vi "Driver.vi"(8 "error in (no error)":errorcluster, 11 "XBoxController":refnum<class "XBoxController.lvclass">) -> (0 "error out":errorcluster)   [LabVIEW 2013]
uses:
  XboxController/XBoxController.lvclass
  DriverXBoxController/DriverXBoxController.lvclass
  DriveMotors/DriveMotors.lvclass
  Shifter/Shifter.lvclass
  XboxController/XBoxController.lvclass/XBoxController.ctl
  Robot Global Data.vi
  <vilib>/Rock Robotics/WPI/Joystick/WPI_JoystickGet.vi
  Commands/DM-SetPower-Command/DM-SetPower-Command.lvclass
panel:
  out "RightPower 2":dbl
  out "LeftPower 2":dbl
  in  "Square Inputs?":bool
  in  "Arcade(T) or Tank(F)":bool=TRUE
  out "Xbox Triggers":T1 {"Right Trigger" scale=0.0..1.0; "Left Trigger" scale=0.0..1.0}
  out "LeftJoystick.Right":dbl(slide) scale=-1.0..1.0
  out "LeftJoystick.Forward":dbl(slide) scale=-1.0..1.0
  out "RightPower":dbl(slide) scale=-1.0..1.0
  out "LeftPower":dbl(slide) scale=-1.0..1.0
  in  "Semaphore Timeout":i32=-1
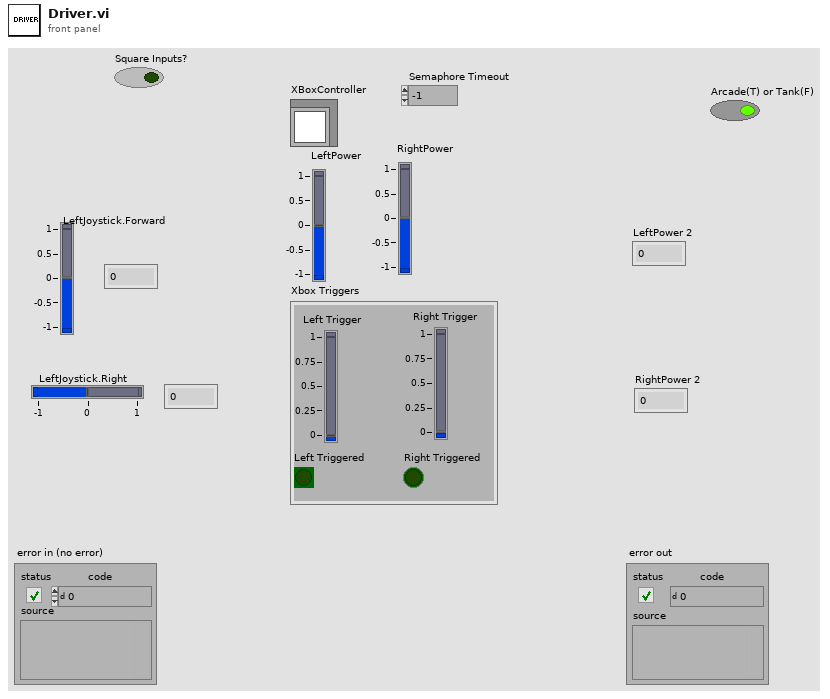
[diagram p1: front panel]
types:
  T1 = cluster{"Left Trigger":dbl, "Right Trigger":dbl, "Left Triggered":bool, "Right Triggered":bool}
  T2 = typedef "XBoxController.lvclass/Xbox Buttons.ctl" = cluster{"RightBumper":bool, "Left Bumper":bool, "Left Joy Down":bool, "Right Joy Down":bool, "Back":bool, "Start":bool, "D-Pad Left":bool, "D-Pad Right":bool, "Y":bool, "B":bool, "A":bool, "X":bool}
  T3 = cluster{"LeftJoystick":cluster{"Forward":dbl, "Right":dbl}, "RightJoystick":cluster{"Forward":dbl, "Right":dbl}}
  T4 = typedef "Semaphore RefNum" = refnum<k1>
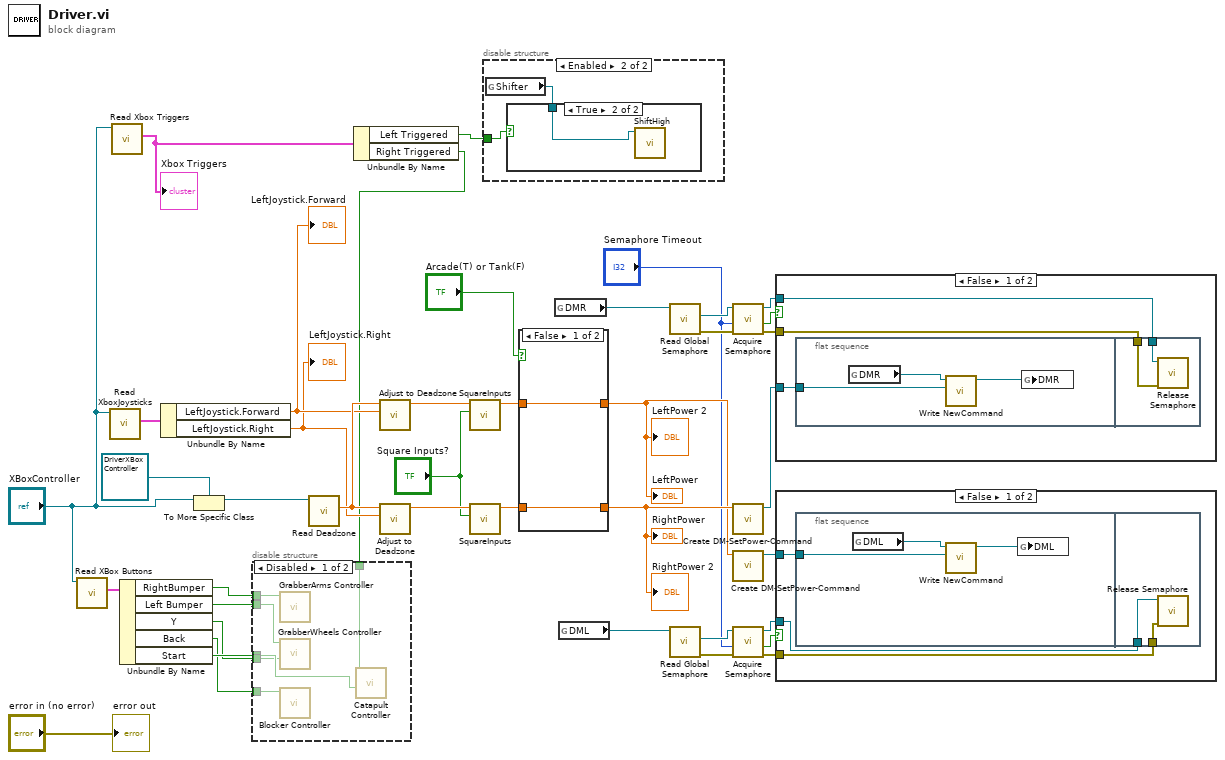
[diagram p0: block diagram]
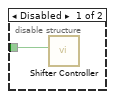
[diagram p2: hidden frame]
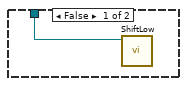
[diagram p3: hidden frame]
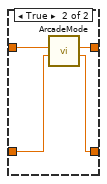
[diagram p5: hidden frame]
diagram:
  n1 = call "Read XBox Buttons.vi"("XBoxController in"="XBoxController") -> ("XBox Buttons"=w8:T2)  [unwired: 8 in, 2 out]
  n2 = call-dynamic "Read XboxJoysticks.vi"("XBoxController in"="XBoxController") -> ("XboxJoysticks"=w40:T3)  [unwired: 8 in, 2 out]
  n3 = call-dynamic "Read Xbox Triggers.vi"("XBoxController in"="XBoxController") -> ("Xbox Triggers"=w38:T1)  [unwired: 8 in, 2 out]
  "Xbox Triggers" <- w38
  n4 = Unbundle By Name(w8) -> ("RightBumper"=w7:bool, "Left Bumper"=w6:bool, "Y"=w4:bool, "Back"=w3:bool, "Start"=w5:bool)
  n5 = Unbundle By Name(w40) -> ("LeftJoystick.Forward"=w11:dbl, "LeftJoystick.Right"=w10:dbl)
  "LeftJoystick.Forward" <- w11
  "LeftJoystick.Right" <- w10
  n6 = To More Specific Class(target class=refnum<class "DriverXBoxController.lvclass"> refnum ("DriverXBoxController.lvclass"), reference="XBoxController") -> (specific class reference=w19:refnum<class "DriverXBoxController.lvclass">)  [unwired: 1 in, 1 out]
  n7 = call-dynamic "Read Deadzone.vi"("DriverXBoxController in"=w19) -> ("Deadzone"=w18:dbl)  [unwired: 8 in, 2 out]
  n8 = Unbundle By Name(w38) -> ("Left Triggered"=w2:bool, "Right Triggered"=w1:bool)
  n9 = disable-structure shown="Disabled" {
    disable-tunnel: w7 -> [w46 _]
    disable-tunnel: w6 -> [w45 _]
    disable-tunnel: w5 -> [w44 _]
    disable-tunnel: w4 -> [w43 _]
    disable-tunnel: w3 -> [w42 _]
    disable-tunnel: w1 -> [w41 _]
    frame Disabled {
      n10 = call "GrabberArms Controller.vi"("Extend GrabberArms"=w46) -> ()  [unwired: 10 in, 1 out]
      n11 = call "GrabberWheels Controller.vi"("GW Spit Out"=w43, "GW Full Speed Pickup"=w45) -> ()  [unwired: 9 in, 1 out]
      n12 = call "Blocker Controller.vi"("Blocker Toggle"=w42) -> ()  [unwired: 11 in]
      n13 = call "Catapult Controller.vi"("De-energize w/out Re-energizing"=w44, "Catapult Trigger"=w41) -> ()  [unwired: 9 in, 1 out]
    }
    frame Enabled {
    }
  }
  n14 = call "Adjust to Deadzone.vi"("Axis Value"=w11, "Deadzone"=w18) -> ("Adjusted Axis Value"=w16:dbl)  [unwired: 9 in]
  n15 = call "Adjust to Deadzone.vi"("Axis Value"=w10, "Deadzone"=w18) -> ("Adjusted Axis Value"=w14:dbl)  [unwired: 9 in]
  n16 = call "SquareInputs.vi"("Square Inputs?"="Square Inputs?", "AxisValueIn"=w16) -> ("AxisValueOut"=w15:dbl)  [unwired: 9 in]
  n17 = call "SquareInputs.vi"("Square Inputs?"="Square Inputs?", "AxisValueIn"=w14) -> ("AxisValueOut"=w13:dbl)  [unwired: 9 in]
  n18 = disable-structure shown="Enabled" {
    disable-tunnel: w2 -> [w47 w48]
    frame Disabled {
      n19 = call "Shifter Controller.vi"("ShiftHigh"=w47) -> ()  [unwired: 11 in]
    }
    frame Enabled {
      n20 = global read "Robot Global Data.vi" "Shifter"() -> (w49:refnum<class "Shifter.lvclass">)
      n21 = case shown="True" w48 {
        tunnel: w49 -> [w50 w51]
        frame False {
          n22 = call-dynamic "ShiftLow.vi"("Shifter in"=w50) -> ()  [unwired: 9 in, 2 out]
        }
        frame True {
          n23 = call-dynamic "ShiftHigh.vi"("Shifter in"=w51) -> ()  [unwired: 9 in, 2 out]
        }
      }
    }
  }
  n24 = case shown="False" "Arcade(T) or Tank(F)" {
    tunnel: [w52 w57] -> w37
    tunnel: [w53 w56] -> w24
    tunnel: w15 -> [w53 w55]
    tunnel: w13 -> [w52 w54]
    frame False {
    }
    frame True {
      n25 = call "ArcadeMode.vi"("RightPower"=w54, "ForwardPower"=w55) -> ("RightPower"=w57:dbl, "LeftPower"=w56:dbl)  [unwired: 8 in]
    }
  }
  "LeftPower" <- w24
  "RightPower" <- w37
  "LeftPower 2" <- w24
  "RightPower 2" <- w37
  n26 = global read "Robot Global Data.vi" "DMR"() -> (w35:refnum<class "DriveMotors.lvclass">)
  n27 = global read "Robot Global Data.vi" "DML"() -> (w31:refnum<class "DriveMotors.lvclass">)
  n28 = call-dynamic "Read Global Semaphore.vi"("System in"=w35) -> ("error out"=w27:errorcluster, "semaphore"=w34:T4)  [unwired: 8 in, 1 out]
  n29 = call-dynamic "Read Global Semaphore.vi"("System in"=w31) -> ("error out"=w28:errorcluster, "semaphore"=w30:T4)  [unwired: 8 in, 1 out]
  n30 = call <vilib>:"Acquire Semaphore.vi"("error in (no error)"=w27, "ms timeout (-1)"="Semaphore Timeout", "semaphore"=w34) -> ("error out"=w26:errorcluster, "timed out"=w33:bool, "semaphore out"=w32:T4)  [unwired: 2 in]
  n31 = call "Create DM-SetPower-Command.vi"("LeftPower"=w37) -> ("DM-SetPower-Command out"=w36:refnum<class "DM-SetPower-Command.lvclass">)  [unwired: 9 in, 1 out]
  n32 = call "Create DM-SetPower-Command.vi"("LeftPower"=w24) -> ("DM-SetPower-Command out"=w23:refnum<class "DM-SetPower-Command.lvclass">)  [unwired: 9 in, 1 out]
  n33 = call <vilib>:"Acquire Semaphore.vi"("error in (no error)"=w28, "ms timeout (-1)"="Semaphore Timeout", "semaphore"=w30) -> ("error out"=w25:errorcluster, "timed out"=w29:bool, "semaphore out"=w22:T4)  [unwired: 2 in]
  n34 = case shown="False" w33 {
    tunnel: w36 -> [w59 _]
    tunnel: w32 -> [w60 _]
    tunnel: w26 -> [w58 _]
    frame False {
      n35 = flat-sequence {
        tunnel: w59 -> [w61]
        tunnel: w60 -> [w65]
        tunnel: w58 -> [w64]
        frame #0 {
          n36 = global read "Robot Global Data.vi" "DMR"() -> (w62:refnum<class "DriveMotors.lvclass">)
          n37 = call-dynamic "Write NewCommand.vi"("Command.lvclass"=w61, "System in"=w62) -> ("System out"=w63:refnum<class "DriveMotors.lvclass">)  [unwired: 8 in, 1 out]
          n38 = global write "Robot Global Data.vi" "DMR"(w63) -> ()
        }
        frame #1 {
          n39 = call <vilib>:"Release Semaphore.vi"("error in (no error)"=w64, "semaphore"=w65) -> ()  [unwired: 4 in, 2 out]
        }
      }
    }
    frame True {
    }
  }
  n40 = case shown="False" w29 {
    tunnel: w25 -> [w68 _]
    tunnel: w23 -> [w67 _]
    tunnel: w22 -> [w66 _]
    frame False {
      n41 = flat-sequence {
        tunnel: w67 -> [w69]
        tunnel: w68 -> [w73]
        tunnel: w66 -> [w72]
        frame #0 {
          n42 = global read "Robot Global Data.vi" "DML"() -> (w70:refnum<class "DriveMotors.lvclass">)
          n43 = call-dynamic "Write NewCommand.vi"("Command.lvclass"=w69, "System in"=w70) -> ("System out"=w71:refnum<class "DriveMotors.lvclass">)  [unwired: 8 in, 1 out]
          n44 = global write "Robot Global Data.vi" "DML"(w71) -> ()
        }
        frame #1 {
          n45 = call <vilib>:"Release Semaphore.vi"("error in (no error)"=w73, "semaphore"=w72) -> ()  [unwired: 4 in, 2 out]
        }
      }
    }
    frame True {
    }
  }
  "error out" <- "error in (no error)"
